vi "turn off and on monitor.vi"(8 "错误输入（无错误）":errorcluster, 11 "Delay Time (s)":dbl=5.0 caption="关闭时间(s)") -> (0 "错误输出":errorcluster)   [LabVIEW 2011]
uses:
  user32.dll
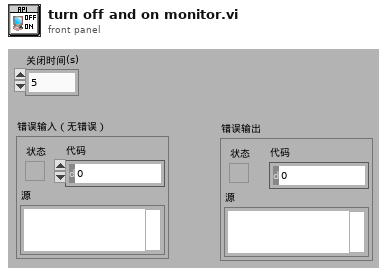
[diagram p1: front panel]
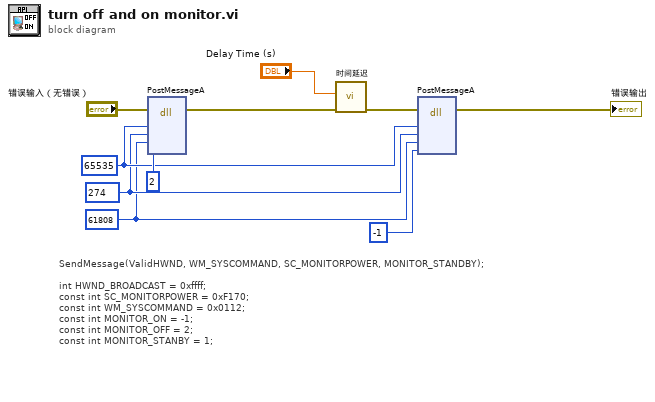
[diagram p0: block diagram]
diagram:
  w3 = 61808 ("wParam")
  w4 = u32 274 ("Msg")
  w5 = 65535 ("hWnd")
  # "SendMessage(ValidHWND, WM_SYSCOMMAND, SC_MONITORPOWER, MONITOR_STANDBY);\n\nint HWND_BROADCAST = 0xffff;\nconst int SC_MONITORPOWER = 0xF170;\nconst int WM_SYSCOMMAND = 0x0112;\nconst int MONITOR_ON = -1;\nconst int MONITOR_OFF = 2;\nconst int MONITOR_STANBY = 1;"
  n1 = dll-call lib="user32.dll" fn="PostMessageA"(error in="错误输入（无错误）", "hWnd"=w5, "Msg"=w4, "wParam"=w3, "lParam"=2) -> (error out=w8:errorcluster)  [unwired: 7 in, 1 out]
  n2 = call "时间延迟"("error in (no error)"=w8, "Delay Time (s)"="Delay Time (s)") -> ("error out"=w9:errorcluster)  [unwired: 9 in]
  n3 = dll-call lib="user32.dll" fn="PostMessageA"(error in=w9, "hWnd"=w5, "Msg"=w4, "wParam"=w3, "lParam"=-1) -> (error out=→"错误输出":errorcluster)  [unwired: 7 in, 1 out]
